vi "proje.vi"() -> ()   [LabVIEW 2021]
uses:
  <vilib>/Instr/_visa.llb/VISA Configure Serial Port (Instr).vi
panel:
  in  "baud rate (9600)":u32=9600
  in  "VISA resource name":refnum<visa-resource-name>
  out "ölçüm mesafesi dýþýnda":bool
  out "ölçüm mesafesi içerisinde":bool
  out "mesafe":string
  in  "stop":bool
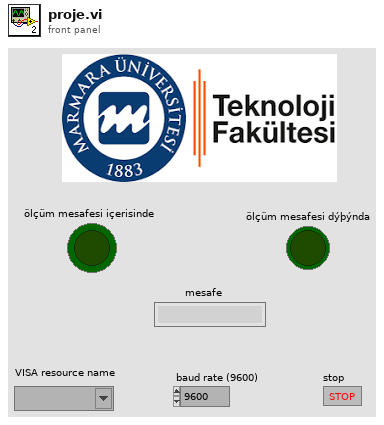
[diagram p1: front panel]
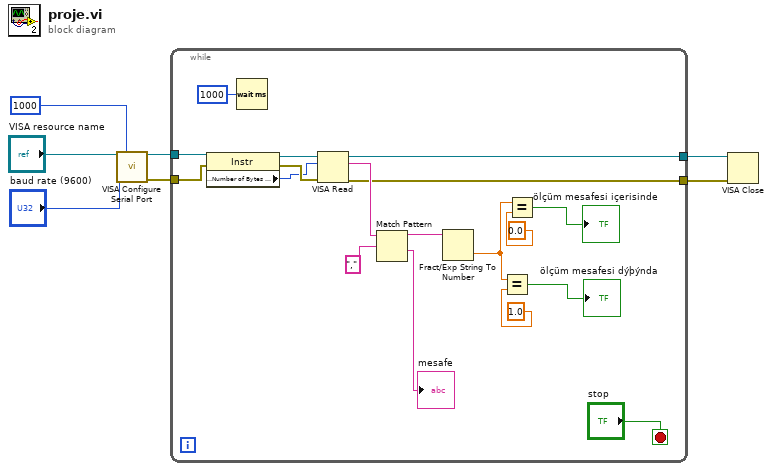
[diagram p0: block diagram]
diagram:
  n1 = call-poly "VISA Configure Serial Port"("VISA resource name"="VISA resource name", "timeout (10sec)"=u32 1000, "baud rate (9600)"="baud rate (9600)") -> ("VISA resource name out"=w6:refnum<visa-resource-name>, "error out"=w5:errorcluster)  [unwired: 11 in]
  n2 = while {
    tunnel: w6 -> [w24]
    tunnel: w5 -> [w23]
    tunnel: [w9] -> w2
    tunnel: [w8] -> w1
    stop <- "stop" stop-if-true
    n3 = property class="Instr"(reference=w24, error in=w23) -> (reference out=w12:refnum<visa-resource-name>, error out=w11:errorcluster, "Serial Settings:Number of Bytes at Serial Port"=w10:u32)
    n4 = Wait (ms)(milliseconds to wait=u32 1000) -> ()  [unwired: 1 out]
    n5 = VISA Read(VISA resource name=w12, byte count=w10, error in (no error)=w11) -> (VISA resource name out=w9:refnum<visa-resource-name>, read buffer=w20:string, error out=w8:errorcluster)  [unwired: 1 out]
    n6 = Match Pattern(string=w20, regular expression=",") -> (before substring=w13:string, after substring=→"mesafe":string)  [unwired: 1 in, 2 out]
    n7 = Fract/Exp String To Number(string=w13) -> (number=w15:dbl)  [unwired: 3 in, 1 out]
    n8 = Equal?(x=w15, y=1.0) -> (x = y?=→"ölçüm mesafesi dýþýnda":bool)
    n9 = Equal?(x=w15, y=0.0) -> (x = y?=→"ölçüm mesafesi içerisinde":bool)
  }
  n10 = VISA Close(VISA resource name=w2, error in (no error)=w1) -> ()  [unwired: 1 out]
